vi "test Standard Application Flow.vi"(8 "error in":errorcluster) -> (0 "error out":errorcluster)   [LabVIEW 2020, in "ase.test.lvlib"]
uses:
  ase.test.lvlib
  ase/ase/Configuration.ctl
  ase/ase/Windows UTF8 Conversion Mode.ctl
  ase/ase/ase.lvclass/ase.ctl
  ase/ase/Trim Whitespace.vi
  ase/ase/Merge Call Library Errors.vi
  ase/ase/Check Shared Library Version.vi
  ase/ase/Start Call.vi/a70fc713-9ee9-4497-bede-7e71c94245f2.vi
  ase/ase/Error Invalid ASE Handle.vi
  ase/ase/Error Internal Library Implementation Error.vi
  <vilib>/Utility/file.llb/Application Directory.vi
  <vilib>/addons/_JKI Toolkits/Caraya/classes/Assert/Assert Not Error.vi
  <vilib>/addons/_JKI Toolkits/Caraya/classes/Assert/Assert Equal Value_Variant.vi
  ase/ase/Wait on Call.vi
  <vilib>/addons/_JKI Toolkits/Caraya/classes/Assert/Assert True.vi
  ase/ase/ase.lvclass
  <vilib>/addons/_JKI Toolkits/Caraya/classes/Assert/Assert.lvclass
  <vilib>/addons/_JKI Toolkits/Caraya/classes/Test/Test.lvclass
panel:
  out "Std Err":string
  out "Std Out":string
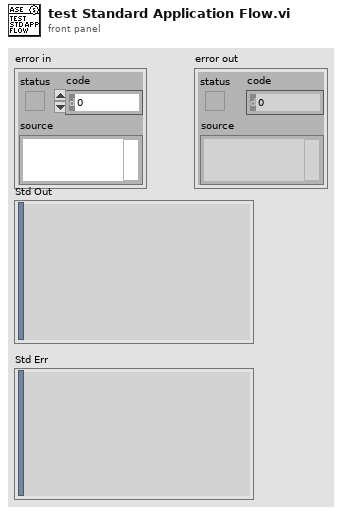
[diagram p1: front panel]
types:
  T1 = cluster{"Remaining StdOut":string, "Remaining StdErr":string}
  T2 = typedef "ase.lvlib/ase.lvclass/Configuration.ctl" = cluster{"Std Out Stream-Split RegExp Pattern":string, "Std Err Stream-Split RegExp Pattern":string, "ID":string, "Windows UTF8 Conversion":T3}
  T3 = typedef "ase.lvlib/ase.lvclass/Windows UTF8 Conversion Mode.ctl" = enum8{"None (Pass Through UTF8)", "To ACP Code Page", "To OEM Code Page"}
  T4 = typedef "ase.lvlib/ase.lvclass/Event References.ctl" = cluster{"Standard Output":refnum<user-event>, "Standard Error":refnum<user-event>, "Did Exit":refnum<user-event>}
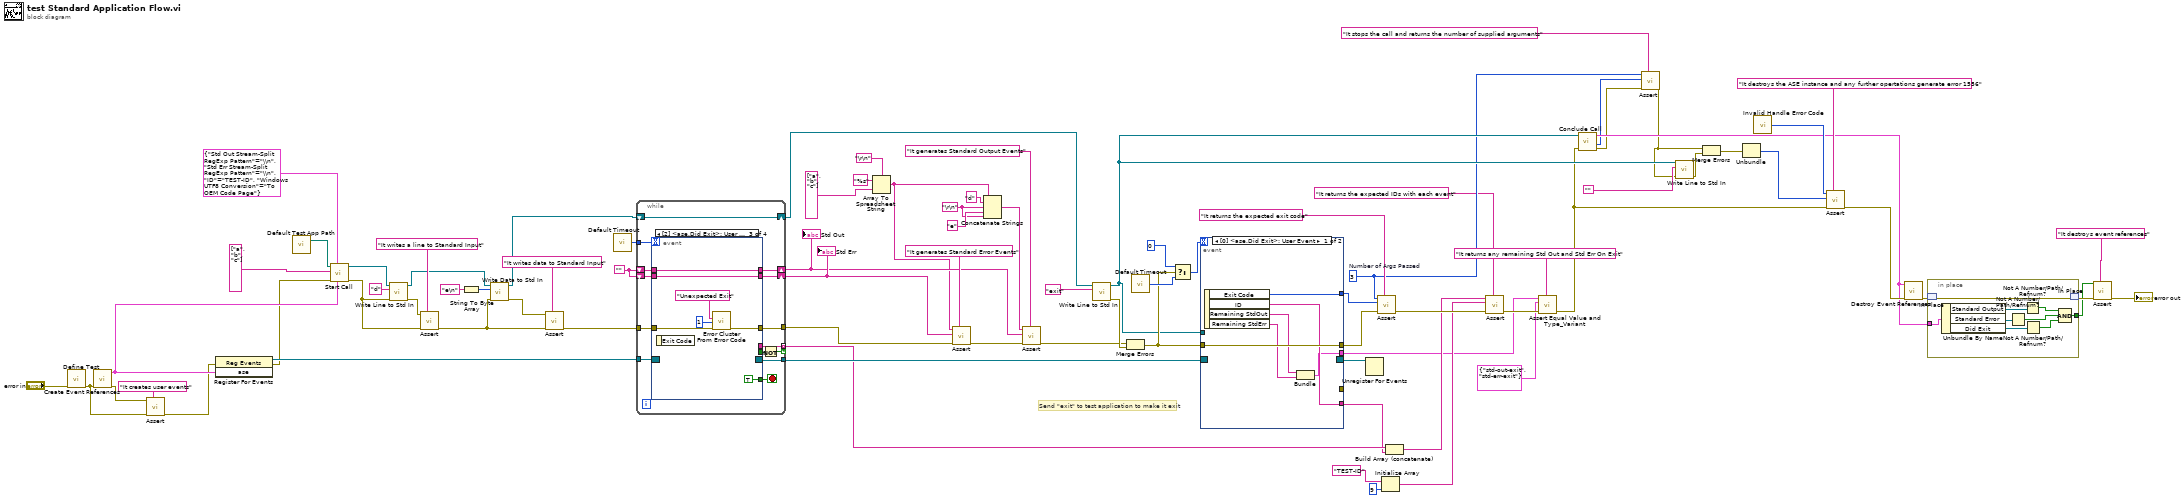
[diagram p0: block diagram]
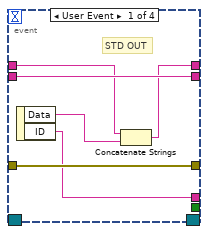
[diagram p2: hidden frame]
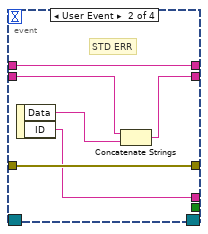
[diagram p3: hidden frame]
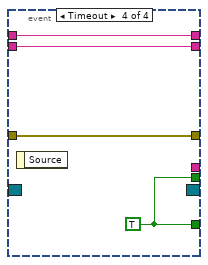
[diagram p4: hidden frame]
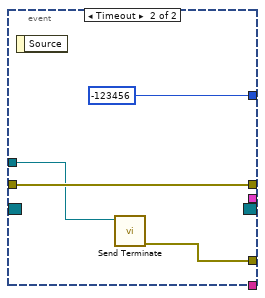
[diagram p5: hidden frame]
diagram:
  w52 = "\r\n"
  w21 = 3  # Number of Args Passed
  w78 = "" ("Empty String Constant")
  # "Send \"exit\" to test application to make it exit"
  n1 = call <vilib>:"Define Test.vi"("error in (no error)"="error in") -> ("error out"=w45:errorcluster)  [unwired: 9 in, 1 out]
  n2 = call "Create Event References.vi"("error in"=w45) -> ("error out"=w44:errorcluster, "ase"=w63:T4)  [unwired: 9 in]
  n3 = call-poly <vilib>:"Assert.vi"("Label"="It creates user events", "error in (no error)"=w45, "Not Error?"=w44) -> ("error out"=w43:errorcluster)  [unwired: 7 in, 1 out]
  n4 = register-events(error in=w43, w63) -> (reference out=w64:refnum<event-registration>, error out=w42:errorcluster)  [unwired: 1 in]
  n5 = call "Default Test App Path.vi"() -> ("Exe Path With Extention"=w7:path)  [unwired: 2 in, 1 out]
  n6 = call "Start Call.vi"("Event References"=w63, "Configuration (Default)"=T2 {"Std Out Stream-Split RegExp Pattern"="\\n", "Std Err Stream-Split RegExp Pattern"="\\n", "ID"="TEST-ID", "Windows UTF8 Conversion"=enum."To OEM Code Page"}, "error in"=w42, "Arguments (Default: Empty)"=string[] ["a", "b", "c"] ("Arguments"), "Executable Path"=w7) -> ("error out"=w51:errorcluster, "New ASE Handle"=w37:refnum<class "ase.lvclass">)  [unwired: 5 in]
  n7 = call "Write Line to Std In .vi"("error in"=w51, "Input"="d", "ASE Handle"=w37) -> ("error out"=w62:errorcluster, "ASE Handle Duplicate"=w35:refnum<class "ase.lvclass">)  [unwired: 6 in, 1 out]
  n8 = call-poly <vilib>:"Assert.vi"("Label"="It writes a line to Standard Input", "error in (no error)"=w51, "Not Error?"=w62) -> ("error out"=w50:errorcluster)  [unwired: 7 in, 1 out]
  n9 = String To Byte Array(string="e\n") -> (unsigned byte array=w58:u8[])
  n10 = call "Write Data to Std In.vi"("error in"=w50, "Data"=w58, "ASE Handle"=w35) -> ("error out"=w61:errorcluster, "ASE Handle Duplicate"=w29:refnum<class "ase.lvclass">)  [unwired: 6 in, 1 out]
  n11 = call-poly <vilib>:"Assert.vi"("Label"="It writes data to Standard Input", "error in (no error)"=w50, "Not Error?"=w61) -> ("error out"=w84:errorcluster)  [unwired: 7 in, 1 out]
  n12 = call "Default Timeout.vi"() -> ("Default Timeout"=w77:i32)
  n13 = while {
    tunnel: w84 -> [w99]
    tunnel: w64 -> [w97]
    tunnel: [w96] -> w70
    shift-right: [w91] -> w56
    shift-left: w78 -> [w94]
    shift-right: [w93] -> w76
    shift-left: w78 -> [w92]
    tunnel: w77 -> [w90]
    tunnel: [w98] -> w10
    shift-right: [w89] -> w28
    shift-left: w29 -> [w89]
    tunnel: [w88] -> w20 mode=indexing if=w86
    stop <- w95 stop-if-true
    n14 = event shown="[2] <ase.Did Exit>: User Event" {
      selector: w97 -> [_ _ _ _]
      dyn-events: [_ _ _ _] -> w96
      timeout: w90 -> [_ _ _ _]
      tunnel: w99 -> [w105 w111 w114 w122]
      tunnel: [w105 w111 w115 w122] -> w98
      tunnel: [_ _ TRUE w119] -> w95
      tunnel: w94 -> [w102 w109 w118 w120]
      tunnel: [w104 w107 w117 w121] -> w93
      tunnel: w92 -> [w104 w108 w117 w121]
      tunnel: [w101 w109 w118 w120] -> w91
      tunnel: [w100 w106 _ _] -> w88
      tunnel: [_ _ _ w119] -> w87
      event User Event {
        # "STD OUT"
        n15 = event-data() -> ("Data"=w103:string, "ID"=w100:string)  [unwired: 1 in]
        n16 = Concatenate Strings(w102, w103) -> (w101:string)
      }
      event User Event {
        # "STD ERR"
        n17 = event-data() -> ("Data"=w110:string, "ID"=w106:string)  [unwired: 1 in]
        n18 = Concatenate Strings(w108, w110) -> (w107:string)
      }
      event User Event {
        n19 = event-data() -> ()  [unwired: 1 in, 1 out]
        n20 = call <vilib>:"Error Cluster From Error Code.vi"("error in (no error)"=w114, "error message (\"\")"="Unexpected Exit" ("error message (\"\")"), "error code (0)"=1) -> ("error out"=w115:errorcluster)  [unwired: 6 in]
      }
      event Timeout {
        w119 = TRUE
        n21 = event-data() -> ()  [unwired: 1 in, 1 out]
      }
    }
    n22 = Not(x=w87) -> (.not. x?=w86:bool)
  }
  "Std Out" <- w56
  "Std Err" <- w76
  n23 = Array To Spreadsheet String(delimiter (Tab)="\r\n", array=string[] ["a", "b", "c"] ("Arguments"), 3:"%s" ("format string")) -> (spreadsheet string=w11:string)
  n24 = call-poly <vilib>:"Assert.vi"("Label"="It generates Standard Error Events", "error in (no error)"=w10, "Y"=w76, "X"=w11) -> ("error out"=w85:errorcluster)  [unwired: 6 in, 1 out]
  n25 = Concatenate Strings(w11, "d" ("string"), w52, "e" ("string"), w52) -> (w53:string)
  n26 = call-poly <vilib>:"Assert.vi"("Label"="It generates Standard Output Events", "error in (no error)"=w85, "Y"=w56, "X"=w53) -> ("error out"=w30:errorcluster)  [unwired: 6 in, 1 out]
  n27 = call "Write Line to Std In .vi"("Input"="exit", "ASE Handle"=w28) -> ("error out"=w49:errorcluster, "ASE Handle Duplicate"=w27:refnum<class "ase.lvclass">)  [unwired: 7 in, 1 out]
  n28 = Merge Errors(w30, w49) -> (w31:errorcluster)
  n29 = call "Default Timeout.vi"() -> ("Default Timeout"=w48:i32)
  n30 = Select(t=0, s=w31, f=w48) -> (s? t:f=w46:i32)
  n31 = event shown="[0] <ase.Did Exit>: User Event" {
    selector: w70 -> [_ _]
    dyn-events: [_ _] -> w69
    timeout: w46 -> [_ _]
    tunnel: w31 -> [w128 w132]
    tunnel: [w128 w132] -> w83
    tunnel: [w127 -123456 ("Exit Code")] -> w67
    tunnel: w27 -> [_ w130]
    tunnel: [_ w129] -> _
    tunnel: [w126 _] -> w19
    tunnel: [w123 _] -> w3
    event User Event {
      n32 = event-data() -> ("Exit Code"=w127:i32, "ID"=w126:string, "Remaining StdOut"=w125:string, "Remaining StdErr"=w124:string)  [unwired: 1 in]
      n33 = Bundle("Remaining StdOut"=w125, "Remaining StdErr"=w124) -> (w123:T1)  [unwired: 1 in]
    }
    event Timeout {
      n34 = event-data() -> ()  [unwired: 1 in, 1 out]
      n35 = call "Send Terminate.vi"("ASE Handle"=w130) -> ("error out"=w129:errorcluster)  [unwired: 8 in, 2 out]
    }
  }
  n36 = Unregister For Events(event registration refnum=w69) -> ()  [unwired: 1 in, 1 out]
  n37 = call-poly <vilib>:"Assert.vi"("Label"="It returns the expected exit code", "error in (no error)"=w83, "Y"=w67, "X"=w21) -> ("error out"=w18:errorcluster)  [unwired: 6 in, 1 out]
  n38 = Initialize Array("TEST-ID" ("ID (Default - Empty String)"), 9 ("dimension size")) -> (w12:string[])
  n39 = Build Array (concatenate)(w20, w19) -> (w15:string[])
  n40 = call-poly <vilib>:"Assert.vi"("Label"="It returns the expected IDs with each event", "error in (no error)"=w18, "Y"=w12, "X"=w15) -> ("error out"=w17:errorcluster)  [unwired: 6 in, 1 out]
  n41 = call <vilib>:"Assert Equal Value and Type_Variant.vi"("Label"="It returns any remaining Std Out and Std Err On Exit", "error in (no error)"=w17, "Y"=T1 {"Remaining StdOut"="std-out-exit", "Remaining StdErr"="std-err-exit"} ("output cluster"), "X"=w3) -> ("error out"=w4:errorcluster)  [unwired: 6 in, 1 out]
  n42 = call "Conclude Call.vi"("error in"=w4, "ASE Handle"=w27) -> ("error out"=w25:errorcluster, "Exit Code"=w23:i32, "Event References"=w26:T4)  [unwired: 7 in]
  n43 = call-poly <vilib>:"Assert.vi"("Label"="It stops the call and returns the number of supplied arguments", "error in (no error)"=w25, "Y"=w23, "X"=w21) -> ("error out"=w24:errorcluster)  [unwired: 6 in, 1 out]
  n44 = call "Write Line to Std In .vi"("error in"=w24, "Input"="", "ASE Handle"=w27) -> ("error out"=w40:errorcluster)  [unwired: 6 in, 2 out]
  n45 = Merge Errors(w24, w40) -> (w39:errorcluster)
  n46 = Unbundle(w39) -> ("code"=w38:i32)  [unwired: 2 out]
  n47 = call "Invalid Handle Error Code.vi"() -> ("Invalid Handle Error"=w32:i32)
  n48 = call-poly <vilib>:"Assert.vi"("Label"="It destroys the ASE instance and any further opertations generate error 1556", "error in (no error)"=w4, "Y"=w38, "X"=w32) -> ("error out"=w33:errorcluster)  [unwired: 6 in, 1 out]
  n49 = call "Destroy Event References.vi"("error in"=w33, "Event References"=w26) -> ("error out"=w82:errorcluster)  [unwired: 9 in]
  n50 = in-place "In Place Element Structure" {
    in-place-border: [w137] -> w65
    in-place-border: w26 -> [w133]
    n51 = in-place-match #1 ("In Place In / Out Element")(w82) -> (w141:errorcluster)
    n52 = Unbundle By Name(w133) -> ("Standard Output"=w136:refnum<user-event>, "Standard Error"=w135:refnum<user-event>, "Did Exit"=w134:refnum<user-event>)
    n53 = Not A Number/Path/Refnum?(number/path/refnum=w135) -> (NaN/Path/Refnum?=w139:bool)
    n54 = Not A Number/Path/Refnum?(number/path/refnum=w136) -> (NaN/Path/Refnum?=w140:bool)
    n55 = Not A Number/Path/Refnum?(number/path/refnum=w134) -> (NaN/Path/Refnum?=w138:bool)
    n56 = Compound Arithmetic op=AND(w140, w139, w138) -> (w137:bool)
    n57 = in-place-match #1 ("In Place In / Out Element")(w141) -> (w81:errorcluster)
  }
  n58 = call-poly <vilib>:"Assert.vi"("Label"="It destroys event references", "error in (no error)"=w81, "True?"=w65) -> ("error out"=→"error out":errorcluster)  [unwired: 7 in, 1 out]
